vi "proc_create.vi"(5 "use stderr":bool, 7 "hide window":bool=TRUE, 8 "error in":errorcluster, 10 "command":string, 11 "folder":string) -> (0 "error out":errorcluster, 3 "process instance handle":u32[](array[numeric]))   [LabVIEW 2011]
doc: "Creates new process, returns its handler. Even if the process instance has returned exit code the handle must be closed by proc_cleanup.vi!\nIf you wish to access to newly craeted proces instance by your own VI's use process instance handle which has following structure (C/C++ style):\n\ntypedef struct{\n HANDLE proc_handle;\n HANDLE main_thread_handle;\n DWORD process_id;\n DWORD thread_id;\n HANDLE stdout_pipe[2];\n HANDLE stdin_pipe[2];\n}TPHndl;\n\nwhere [1] ends of the pipes are assigned to the new process instance and [0] ends are accessible from the caller (use these to communicate)."
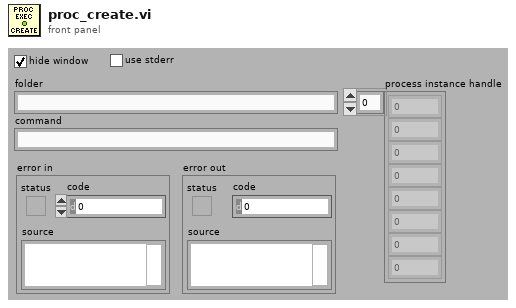
[diagram p1: front panel]
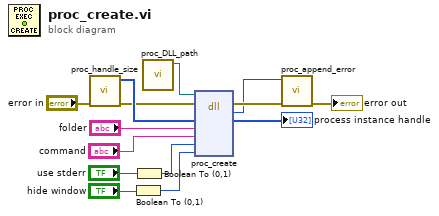
[diagram p0: block diagram]
diagram:
  n1 = call "proc_handle_size.vi"("error in"="error in") -> ("error out"=w3:errorcluster, "new instance handle"=w13:u32[])  [unwired: 8 in, 1 out]
  n2 = Boolean To (0,1)(Boolean="hide window") -> (0, 1=w9:i16)
  n3 = Boolean To (0,1)(Boolean="use stderr") -> (0, 1=w2:i16)
  n4 = call "proc_DLL_path.vi"() -> ("path out"=w14:path)  [unwired: 10 in, 1 out]
  n5 = dll-call lib="lv_proc.dll" fn="proc_create"(path in=w14, error in=w3, "proc"=w13, "folder"="folder", "command"="command", "use_stderr"=w2, "hide_window"=w9) -> (error out=w7:errorcluster, "error"=w5:i32, "proc"=→"process instance handle":u32[])  [unwired: 5 in, 1 out]
  n6 = call "proc_append_error.vi"("error in"=w7, "code in"=w5) -> ("error out"=→"error out":errorcluster)  [unwired: 8 in, 1 out]
